vi "JSON to LabVIEW.vi"(7 "Default Value":variant, 8 "error in (no error)":errorcluster, 11 "JSON Value":T1) -> (0 "error out":errorcluster, 3 "LV Value":variant)   [LabVIEW 2015, in "JSON.lvlib"]
uses:
  JSON.lvlib
  JSON Value.ctl
  Value.ctl
  Value Type.ctl
  Name-Value Pair.ctl
  <vilib>/Utility/Data Type/NI_Data Type.lvlib
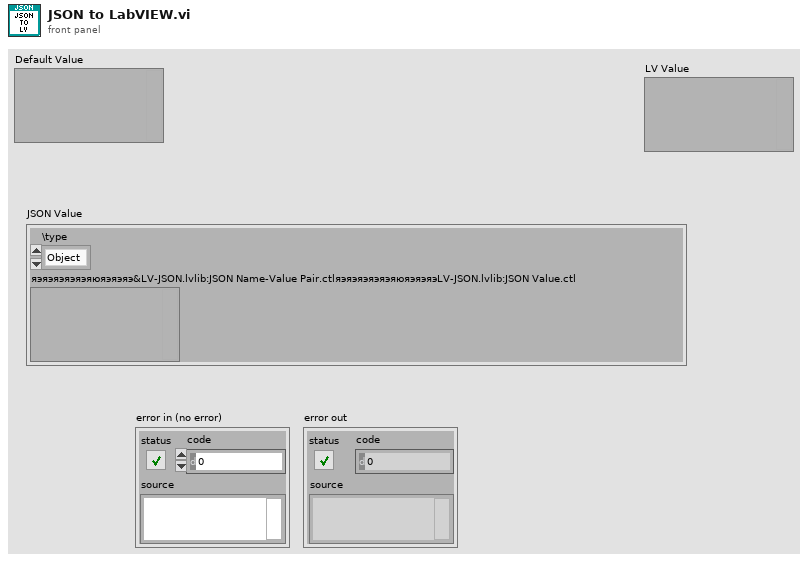
[diagram p1: front panel]
types:
  T1 = typedef "JSON.lvlib/JSON Value.ctl" = cluster{"\\type":enum16{"Object", "Array", "String", "Number", "Boolean", "Null"}, "яэяэяэяэяэяюяэяэяэ&LV-JSON.lvlib:JSON Name-Value Pair.ctlяэяэяэяэяэяюяэяэяэLV-JSON.lvlib:JSON Value.ctl":variant}
  T2 = typedef "JSON.lvlib/Value.ctl" = cluster{"Type":T3, "Value":variant}
  T3 = typedef "JSON.lvlib/Value Type.ctl" = enum16{"Object", "Array", "String", "Number", "Boolean", "Null"}
  T4 = typedef "JSON.lvlib/Name-Value Pair.ctl" = cluster{"Name":string, "Value":T2}
  T5 = typedef "NI_Data Type.lvlib/Data Type.ctl" = enum8{"Invalid Type", "Void", "I8", "I16", "I32", "I64", "U8", "U16", "U32", "U64", "Single Float", "Double Float", "Extended Float", "Single Complex", "Double Complex", "Extended Complex", "Enum U8", "Enum U16", "Enum U32", "Enum U64", "Single Float With Unit", "Double Float With Unit", "Extended Float With Unit", "Single Complex with Unit", "Double Complex with Unit", "Extended Complex with Unit", "Boolean", "String", "Path", "Picture", "Tag", "Array", "Cluster", "Variant", "LV Variant", "Waveform", "Timestamp", "Digital Waveform", "Digital Data", "ExpressData", "Refnum", "External Data", "VI", "Poly VI", "LabVIEW Class Instance", "Fixed Point"}
  T6 = typedef "NI_Data Type.lvlib/Memory Info.ctl" = cluster{"Type":T7, "Size":u32}
  T7 = typedef "NI_Data Type.lvlib/Memory Type.ctl" = enum16{"Variable", "Fixed", "Bounded"}
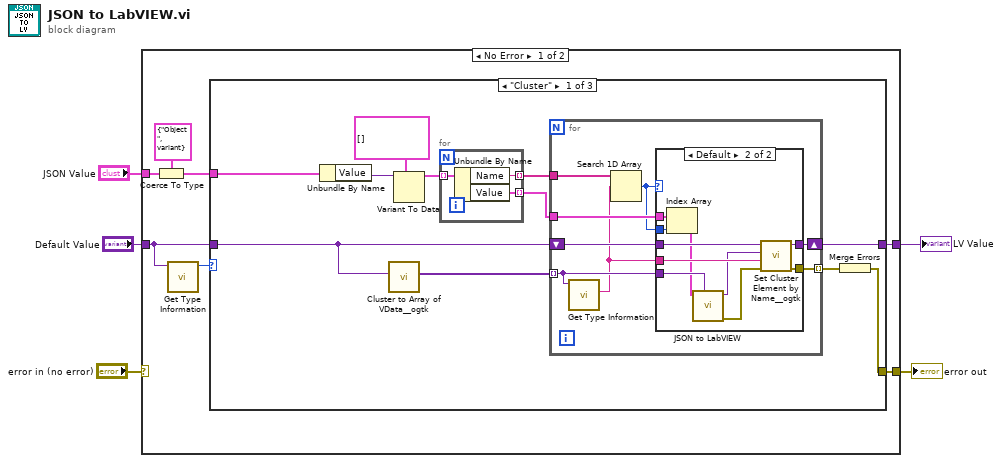
[diagram p0: block diagram]
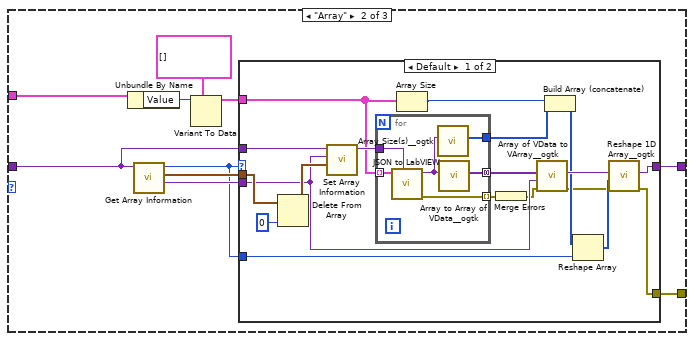
[diagram p3: hidden frame]
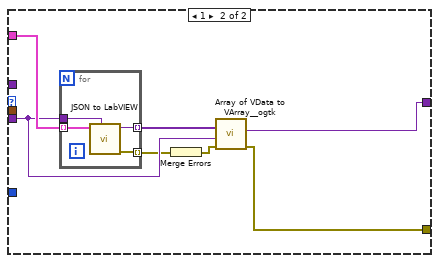
[diagram p4: hidden frame]
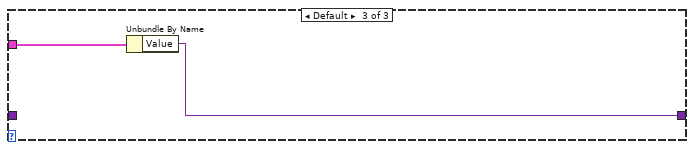
[diagram p5: hidden frame]
diagram:
  n1 = case shown="No Error" "error in (no error)" {
    selector: "error in (no error)" -> [_ w94]
    tunnel: "Default Value" -> [w11 _]
    tunnel: [w10 _] -> w4
    tunnel: "JSON Value" -> [w9 _]
    tunnel: [w6 w94] -> w1
    frame No Error {
      n2 = Coerce To Type(0:w9, 1:T2 {"Type"=enum."Object", "Value"=variant} ("type")) -> (2:w8:T2)
      n3 = call <vilib>:"Get Type Information.vi"("Variant"=w11) -> ("Type"=w12:T5)  [unwired: 6 in, 4 out]
      n4 = case shown="\"Cluster\"" w12 {
        tunnel: w8 -> [w23 w55 w93]
        tunnel: w11 -> [w14 w51 _]
        tunnel: [w17 w48 w92] -> w10
        tunnel: [w15 w46 _] -> w6
        frame "Cluster" {
          n5 = Unbundle By Name(w23) -> ("Value"=w22:variant)
          n6 = call <userlib>:"Cluster to Array of VData__ogtk.vi"("Cluster"=w14) -> ("Array of VData"=w13:variant[])  [unwired: 9 in, 1 out]
          n7 = Variant To Data(type=T4[] [], Variant=w22) -> (data=w19:T4[])  [unwired: 1 in, 1 out]
          n8 = for {
            tunnel: w19 -> [w26] mode=indexing
            tunnel: [w25] -> w20 mode=indexing
            tunnel: [w24] -> w18 mode=indexing
            n9 = Unbundle By Name(w26) -> ("Name"=w25:string, "Value"=w24:T2)
          }
          n10 = for {
            tunnel: w13 -> [w31] mode=indexing
            tunnel: w20 -> [w34]
            tunnel: w18 -> [w33]
            shift-right: [w32] -> w17
            shift-left: w14 -> [w30]
            tunnel: [w27] -> w16 mode=indexing
            n11 = call <vilib>:"Get Type Information.vi"("Variant"=w31) -> ("Name"=w29:string)  [unwired: 6 in, 4 out]
            n12 = Search 1D Array(1D array=w34, element=w29) -> (index of element=w28:i32)  [unwired: 1 in]
            n13 = case shown="Default" w28 {
              tunnel: w33 -> [_ w45]
              tunnel: w28 -> [_ w44]
              tunnel: [w35 w43] -> w32
              tunnel: w31 -> [_ w42]
              tunnel: w30 -> [w35 w41]
              tunnel: w29 -> [_ w40]
              tunnel: [_ w36] -> w27
              frame -1 {
              }
              frame Default {
                n14 = Index Array(array=w45, index=w44) -> (element=w39:T2)
                n15 = call "JSON to LabVIEW.vi"("Default Value"=w42, "JSON Value"=w39) -> ("error out"=w37:errorcluster, "LV Value"=w38:variant)  [unwired: 8 in]
                n16 = call <userlib>:"Set Cluster Element by Name__ogtk.vi"("error in (no error)"=w37, "Element Name (\"\": New Element Data Name)"=w40, "New Element Value"=w38, "Cluster"=w41) -> ("error out"=w36:errorcluster, "VCluster out"=w43:variant)  [unwired: 5 in, 1 out]
              }
            }
          }
          n17 = Merge Errors(w16) -> (w15:errorcluster)
        }
        frame "Array" {
          n18 = Unbundle By Name(w55) -> ("Value"=w54:variant)
          n19 = call <vilib>:"Get Array Information.vi"("Variant"=w51) -> ("Array Element Data Type"=w52:variant, "Array Lengths"=w50:T6[], "Number of Dimensions"=w47:i32)  [unwired: 7 in, 1 out]
          n20 = Variant To Data(type=T2[] [], Variant=w54) -> (data=w49:T2[])  [unwired: 1 in, 1 out]
          n21 = case shown="Default" w47 {
            tunnel: w52 -> [w63 w85]
            tunnel: w51 -> [w74 _]
            tunnel: w50 -> [w73 _]
            tunnel: w49 -> [w69 w87]
            tunnel: [w66 w84] -> w48
            tunnel: w47 -> [w62 _]
            tunnel: [w56 w81] -> w46
            frame Default {
              n22 = Delete From Array(array=w73, index=0) -> (array with subset deleted=w71:T6[])  [unwired: 1 in, 1 out]
              n23 = call <vilib>:"Set Array Information.vi"("Array Lengths"=w71, "Array Element"=w63, "Variant in"=w74) -> ("Variant out"=w70:variant)  [unwired: 7 in, 1 out]
              n24 = for {
                tunnel: w70 -> [w80]
                tunnel: w69 -> [w77] mode=indexing
                tunnel: [w79] -> w67
                tunnel: [w78] -> w65 mode=concatenating
                tunnel: [w75] -> w59 mode=indexing
                n25 = call "JSON to LabVIEW.vi"("Default Value"=w80, "JSON Value"=w77) -> ("error out"=w75:errorcluster, "LV Value"=w76:variant)  [unwired: 8 in]
                n26 = call <userlib>:"Array Size(s)__ogtk.vi"("Array"=w76) -> ("Size(s)"=w79:u32[])  [unwired: 8 in, 2 out]
                n27 = call <userlib>:"Array to Array of VData__ogtk.vi"("MultiD Array"=w76) -> ("1D Array of Variants"=w78:variant[])  [unwired: 9 in, 1 out]
              }
              n28 = Array Size(array=w69) -> (size(s)=w68:i32)
              n29 = Merge Errors(w59) -> (w58:errorcluster)
              n30 = call <userlib>:"Array of VData to VArray__ogtk.vi"("error in (no error)"=w58, "Element Type (when empty)"=w63, "1D Array of VData"=w65) -> ("error out"=w57:errorcluster, "VArray"=w64:variant)  [unwired: 7 in]
              n31 = Build Array (concatenate)(w68, w67) -> (w61:u32[])
              n32 = Reshape Array(w61, w62) -> (w60:u32[])
              n33 = call <userlib>:"Reshape 1D Array__ogtk.vi"("error in (no error)"=w57, "Size(s)"=w60, "1D Array"=w64) -> ("error out"=w56:errorcluster, "Reshaped VArray"=w66:variant)  [unwired: 7 in]
            }
            frame 1 {
              n34 = for {
                tunnel: w85 -> [w91]
                tunnel: w87 -> [w90] mode=indexing
                tunnel: [w89] -> w86 mode=indexing
                tunnel: [w88] -> w83 mode=indexing
                n35 = call "JSON to LabVIEW.vi"("Default Value"=w91, "JSON Value"=w90) -> ("error out"=w88:errorcluster, "LV Value"=w89:variant)  [unwired: 8 in]
              }
              n36 = Merge Errors(w83) -> (w82:errorcluster)
              n37 = call <userlib>:"Array of VData to VArray__ogtk.vi"("error in (no error)"=w82, "Element Type (when empty)"=w85, "1D Array of VData"=w86) -> ("error out"=w81:errorcluster, "VArray"=w84:variant)  [unwired: 7 in]
            }
          }
        }
        frame Default {
          n38 = Unbundle By Name(w93) -> ("Value"=w92:variant)
        }
      }
    }
    frame Error {
    }
  }
  "LV Value" <- w4
  "error out" <- w1
